vi "3 dof inverse.vi"() -> ()   [LabVIEW 2021]
panel:
  in  "Parameters of 3 DOF":T1={"l1"=230.59, "l2"=112.96, "phi (rad)"=112.96, "l3"=112.96, "X2"=0.0, "Y2"=0.0} caption="Parameters of Delta Robot"
  out "Motor angles":T2
  # "Definitions about the Inputs of inverse Kinematics :"
  # "X2 and Y2  represents the posions  of 3 DOF."
  # "l1 and l2 and l3 respresents links length."
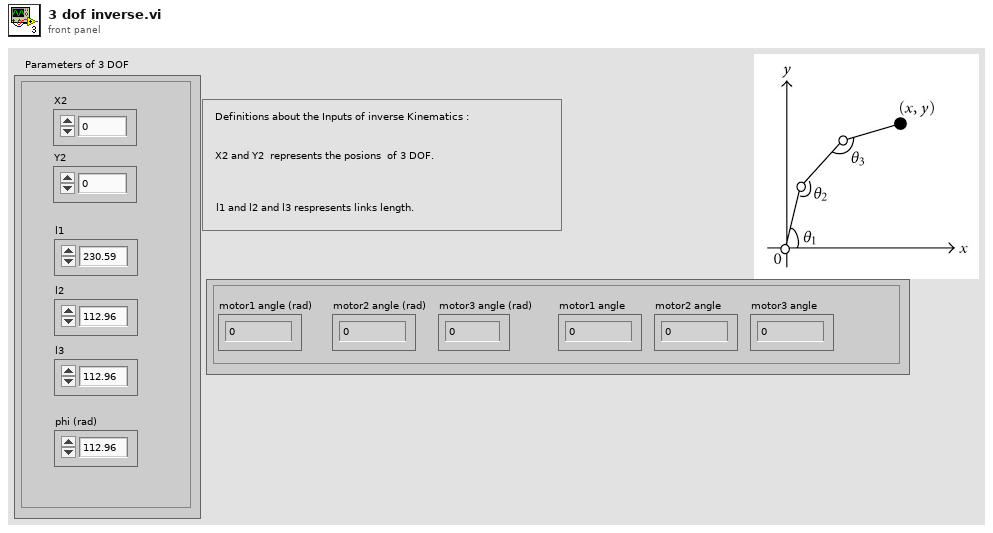
[diagram p1: front panel]
types:
  T1 = cluster{"l1":dbl, "l2":dbl, "phi (rad)":dbl, "l3":dbl, "X2":dbl, "Y2":dbl}
  T2 = cluster{"x":dbl, "y":dbl, "x 2":dbl, "y 2":dbl, "x 3":dbl, "y 3":dbl}
  T3 = cluster{"theta1":dbl, "theta2":dbl, "theta3":dbl, "theta1_dg":dbl, "theta2_dg":dbl, "theta3_dg":dbl}
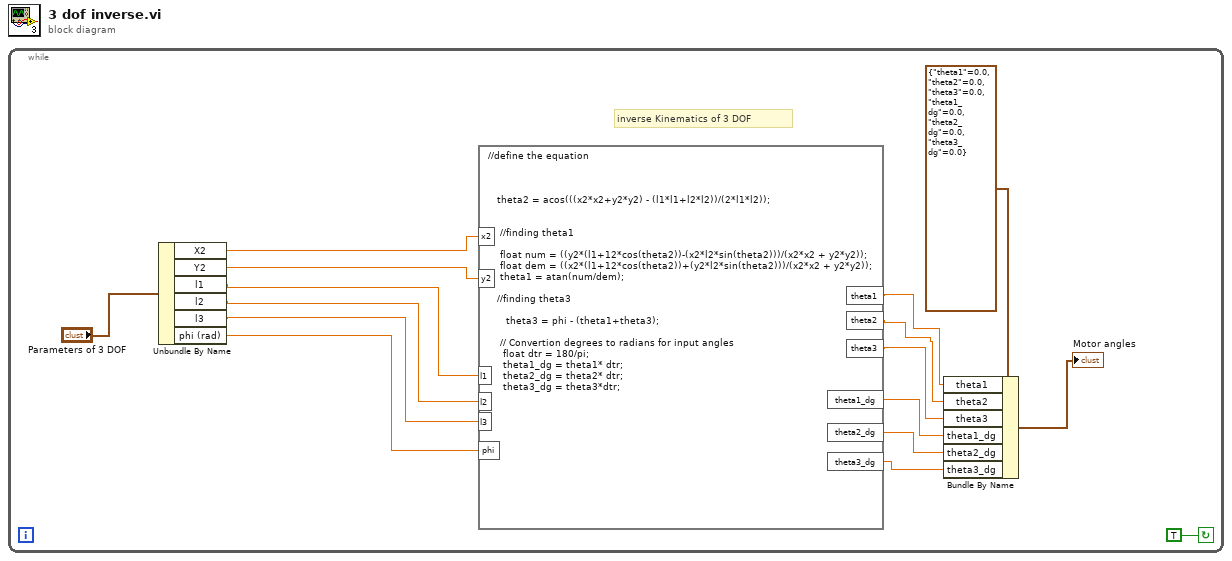
[diagram p0: block diagram]
diagram:
  n1 = while {
    stop <- TRUE continue-if-true
    # "inverse Kinematics of 3 DOF"
    n2 = Unbundle By Name "Unbundle By Name"("Parameters of 3 DOF") -> ("X2"=w14:dbl, "Y2"=w13:dbl, "l1"=w12:dbl, "l2"=w11:dbl, "l3"=w10:dbl, "phi (rad)"=w9:dbl)
    n3 = formula code="//define the equation\n   \n\n  \n   theta2 = acos(((x2*x2+y2*y2) - (l1*l1+l2*l2))/(2*l1*l2)); \n \n    \n    //finding theta1\n\n    float num = ((y2*(l1+12*cos(theta2))-(x2*l2*sin(theta2)))/(x2*x2 + y2*y2));\n    float dem = ((x2*(l1+12*cos(theta2))+(y2*l2*sin(theta2)))/(x2*x2 + y2*y2));\n    theta1 = atan(num/dem);\n    \n   //finding theta3\n   \n      theta3 = phi - (theta1+theta3);\n\n    // Convertion degrees to radians for input angles\n     float dtr = 180/pi;\n     theta1_dg = theta1* dtr;\n     theta2_dg = theta2* dtr;\n     theta3_dg = theta3*dtr;"("l1"=w12, "l2"=w11, "phi"=w9, "l3"=w10, "x2"=w14, "y2"=w13) -> ("theta1"=w7:dbl, "theta2"=w6:dbl, "theta1_dg"=w4:dbl, "theta2_dg"=w3:dbl, "theta3"=w5:dbl, "theta3_dg"=w2:dbl)
    n4 = Bundle By Name(cluster=T3 {"theta1"=0.0, "theta2"=0.0, "theta3"=0.0, "theta1_dg"=0.0, "theta2_dg"=0.0, "theta3_dg"=0.0}, "theta1"=w7, "theta2"=w6, "theta3"=w5, "theta1_dg"=w4, "theta2_dg"=w3, "theta3_dg"=w2) -> (→"Motor angles":T3)
  }
